vi "icListen 4 Metadata.vi"() -> ()   [LabVIEW 2020, in "PAM Library.lvlib"]
uses:
  PAM Library.lvlib
panel:
  out "icListen 4 Metadata":T1 {"Temperature" format="%#_3g"; "Humidity" format="%_3f"}
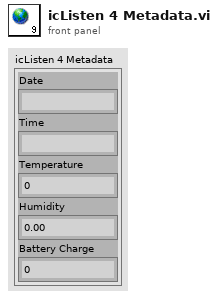
[diagram p1: front panel]
types:
  T1 = cluster{"Date":string, "Time":string, "Temperature":dbl, "Humidity":dbl, "Battery Charge":i32}
diagram:
